vi "ep_Park Demodulation.vi"(8 "error in (no error)":errorcluster, 9 "phase C":dbl[](array[numeric]), 10 "phase B":dbl[](array[numeric]), 11 "phase A":dbl[](array[numeric])) -> (0 "error out":errorcluster, 3 "demodulated signal":dbl[](array[numeric]))   [LabVIEW 2014, in "NI_EP_Motor Monitoring.lvlib"]
uses:
  <vilib>/addons/Electrical Power/Motor Monitoring/NI_EP_Motor Monitoring.lvlib
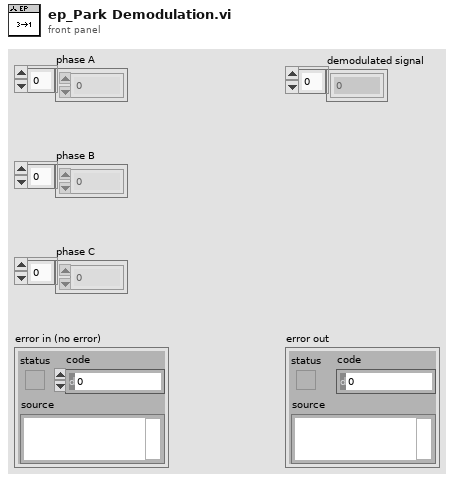
[diagram p1: front panel]
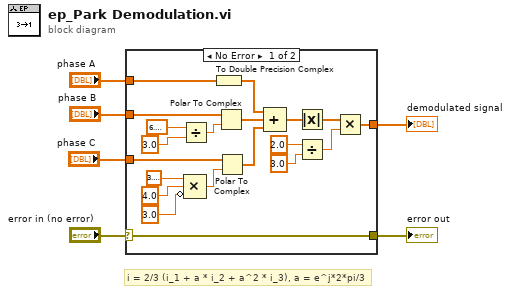
[diagram p0: block diagram]
diagram:
  # "i = 2/3 (i_1 + a * i_2 + a^2 * i_3), a = e^j*2*pi/3"
  n1 = case shown="No Error" "error in (no error)" {
    selector: "error in (no error)" -> [w26 w27]
    tunnel: "phase A" -> [w22 _]
    tunnel: "phase C" -> [w12 _]
    tunnel: "phase B" -> [w20 _]
    tunnel: [w7 _] -> w3
    tunnel: [w26 w27] -> w1
    frame No Error {
      n2 = Divide(x=6.283185307179586, y=3.0) -> (x/y=w19:dbl)
      n3 = Compound Arithmetic op=MULTIPLY(3.141592653589793, 4.0 ("y"), invert 3.0 ("y")) -> (w13:dbl)
      n4 = To Double Precision Complex(1:w22) -> (0:w21:cdb[])
      n5 = Polar To Complex(1:w19, 2:w20) -> (0:w14:cdb[])
      n6 = Polar To Complex(1:w13, 2:w12) -> (0:w11:cdb[])
      n7 = Compound Arithmetic op=ADD(w21, w14, w11) -> (w15:cdb[])
      n8 = Absolute Value(x=w15) -> (abs(x)=w9:dbl[])
      n9 = Divide(x=2.0 ("y"), y=3.0) -> (x/y=w8:dbl)
      n10 = Multiply(x=w9, y=w8) -> (x*y=w7:dbl[])
    }
    frame Error {
    }
  }
  "demodulated signal" <- w3
  "error out" <- w1
